vi "Agilent 428X Series Compensation Application.vi"(0 "VISA resource name":refnum<visa-resource-name>, 5 "Freq Value (Hz)(1.0 kHz)":dbl=1000.0 min=20.0 max=30000000.0 step=10.0 format="%.4e", 7 "Voltage Level (V)(1.0V)":dbl=1.0 min=0.0 max=20.0 step=0.1 format="%.4f", 9 "Imp Type (0: CPD)":u32(ring) items=["CPD", "CPQ", "CPG", "CPRP", "CSD", "CSQ", "CSRS", "LPQ", "LPD", "LPG", "LPRP", "LSD", "LSQ", "LSRS", "RX", "ZTD", "ZTR", "GB", "YTD", "YTR"], 11 "error in (no error)":errorcluster, 12 "Open (F:OFF)":bool, 13 "Short (F:OFF)":bool) -> (4 "VISA resource name out":refnum<visa-resource-name>, 6 "Primary Value":dbl format="%^.4e", 8 "Secondary Value":dbl format="%^.4e", 10 "Data Status":bool=TRUE, 15 "error out":errorcluster)   [LabVIEW 2015]
doc: "This VI is an example of how to use the HP428XA subVIs programmatically. This VI first configures a measurement, sets triggering, do the compensation for the instrument, and then takes measurements.\n\nWARNING: \nThis VI contains a subVI with a pop up dialog box it will require \nmodification if you wish to be able to use this VI without user intervention.\n\nThis function demonstrate one type of impedance measurement that can be made with the HP428XA and it accessories. In this example a 220 pF ceramic capacitor will be measured under the following conditions.\n\n DUT:\n 220 pF ceramic capacitor\n (HP Part Number 0160-4812)\n\n Measurement Conditions: \n \n Function: Cp-D\n Frequency: 1.0 MHz\n Test Signal Level: 1.0 V\n \n Equipment Required:\n\n HP 16047C Test Fixture\n Shorting bar (HP Part Number 5000-4226) or equivalent\n\nNote:\nFor more details see to the operation manual in Chapter 3."
uses:
  <instrlib>/Agilent 428X Series/Agilent 428X Series.lvlib
panel:
  # "© Copyright 1997 National Instruments Corporation.  All Rights Reserved."
  # "© Copyright 2005 National Instruments Corporation.  All Rights Reserved."
  # "HP 4284A"
  # "True\nFalse"
  # "True\nFalse"
  # "WARNING:  \nThis VI contains a subVI with a pop up dialog box it will require \nmodification if you wish to be able to use this VI without user intervention."
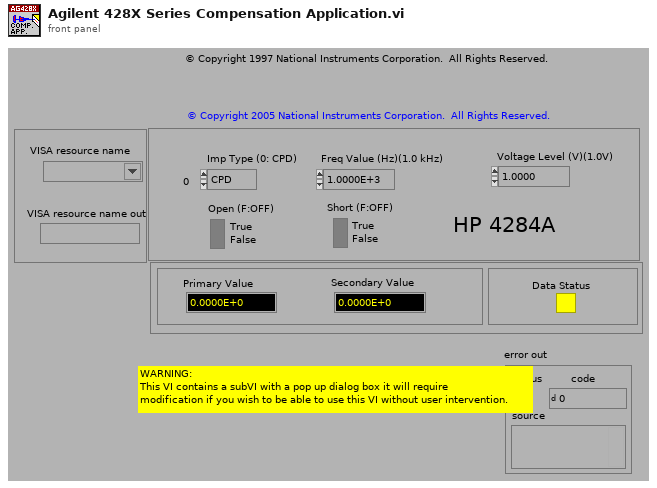
[diagram p1: front panel]
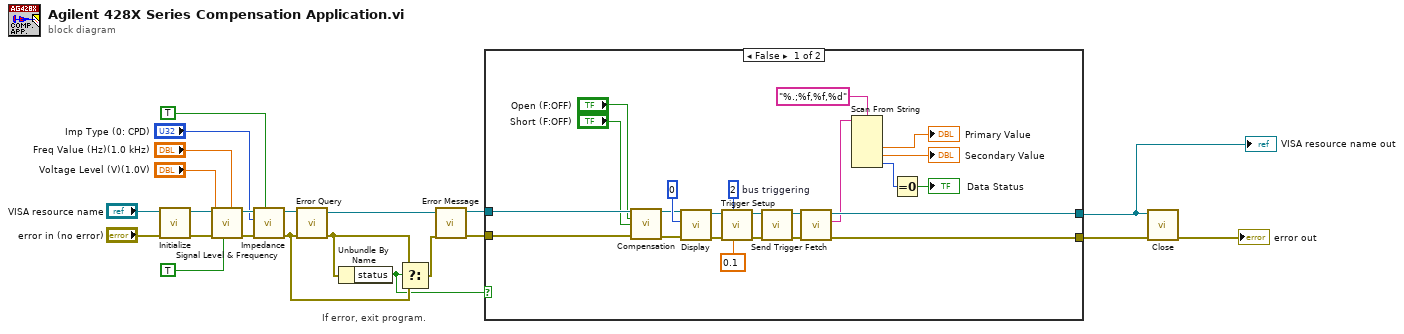
[diagram p0: block diagram]
diagram:
  # "If error, exit program."
  n1 = call <instrlib>:"Initialize.vi"("error in (no error)"="error in (no error)", "VISA resource name"="VISA resource name") -> ("error out"=w4:errorcluster, "VISA resource name out"=w6:refnum<visa-resource-name>)  [unwired: 8 in]
  n2 = call <instrlib>:"Signal Level & Frequency.vi"("Frequency Value (Hz) (100KHz)"="Freq Value (Hz)(1.0 kHz)", "Oscillator Select (T: Voltage)"=TRUE, "error in (no error)"=w4, "Voltage Level (V) (5mV)"="Voltage Level (V)(1.0V)", "VISA resource name"=w6) -> ("error out"=w21:errorcluster, "VISA resource name out"=w22:refnum<visa-resource-name>)  [unwired: 5 in]
  n3 = call <instrlib>:"Impedance.vi"("Auto Range (F: Off)"=TRUE ("Auto Range (On:T)"), "error in (no error)"=w21, "Imp Type (0: CPD)"="Imp Type (0: CPD)", "VISA resource name"=w22) -> ("error out"=w15:errorcluster, "VISA resource name out"=w14:refnum<visa-resource-name>)  [unwired: 6 in]
  n4 = call <instrlib>:"Error Query.vi"("error in (no error)"=w15, "VISA resource name"=w14) -> ("error out"=w13:errorcluster, "VISA resource name out"=w10:refnum<visa-resource-name>)  [unwired: 6 in, 2 out]
  n5 = Unbundle By Name(w13) -> ("status"=w12:bool)
  n6 = Select(t=w13, s=w12, f=w15) -> (s? t:f=w11:errorcluster)
  n7 = call <instrlib>:"Error Message.vi"("error in (no error)"=w11, "VISA resource name"=w10) -> ("error out"=w9:errorcluster, "VISA resource name out"=w8:refnum<visa-resource-name>)  [unwired: 5 in, 3 out]
  n8 = case shown="False" w12 {
    tunnel: w9 -> [w27 w46]
    tunnel: w8 -> [w28 w47]
    tunnel: [w45 w47] -> w3
    tunnel: [w44 w46] -> w1
    frame False {
      w37 = u32 2  # bus triggering
      n9 = call <instrlib>:"Compensation.VI"("VISA resource name"=w28, "OPEN (F:OFF)"="Open (F:OFF)", "SHORT (F:OFF)"="Short (F:OFF)", "error in (no error)"=w27) -> ("VISA resource name out"=w29:refnum<visa-resource-name>, "error out"=w30:errorcluster)  [unwired: 10 in]
      n10 = call <instrlib>:"Display.vi"("error in (no error)"=w30, "Display Page (0: Measurement)"=u32 0 ("Display Page (Measurment:0)"), "VISA resource name"=w29) -> ("error out"=w35:errorcluster, "VISA resource name out"=w31:refnum<visa-resource-name>)  [unwired: 7 in]
      n11 = call <instrlib>:"Trigger Setup.vi"("Delay Value (s) (0.0)"=0.1, "Trigger Source (0: Internal)"=w37, "error in (no error)"=w35, "VISA resource name"=w31) -> ("error out"=w34:errorcluster, "VISA resource name out"=w32:refnum<visa-resource-name>)  [unwired: 6 in]
      n12 = call <instrlib>:"Send Trigger.vi"("error in (no error)"=w34, "VISA resource name"=w32) -> ("error out"=w42:errorcluster, "VISA resource name out"=w33:refnum<visa-resource-name>)  [unwired: 8 in]
      n13 = call <instrlib>:"Fetch.vi"("error in (no error)"=w42, "VISA resource name"=w33) -> ("error out"=w44:errorcluster, "Returned Data"=w38:string, "VISA resource name out"=w45:refnum<visa-resource-name>)  [unwired: 7 in]
      n14 = Scan From String(format string="%.;%f,%f,%d", input string=w38) -> (output 1=→"Primary Value":dbl, output 2=→"Secondary Value":dbl, output 3=w41:i32)  [unwired: 5 in, 3 out]
      n15 = Equal To 0?(x=w41) -> (x = 0?=→"Data Status":bool)
    }
    frame True {
    }
  }
  "VISA resource name out" <- w3
  n16 = call <instrlib>:"Close.vi"("error in (no error)"=w1, "VISA resource name"=w3) -> ("error out"=→"error out":errorcluster)  [unwired: 9 in]
